vi "FGV_Chrono.vi"(7 "FGV_state":T2, 8 "error in":errorcluster caption="entrée d'erreur", 10 "Taget Time":dbl format="%#_g s") -> (0 "error out":errorcluster caption="sortie d'erreur", 3 "Local":T1 {"Countdown" format="%#_g s"; "Previous Pause TimeTime" format="%#_g s"; "Pause TimeTime" format="%#_g s"; "Time" format="%#_g s"})   [LabVIEW 2020]
doc: "FGV chrono"
uses:
  Controls/Ctrl_states.ctl
  Controls/Ctrl_Local_FGV_Time.ctl
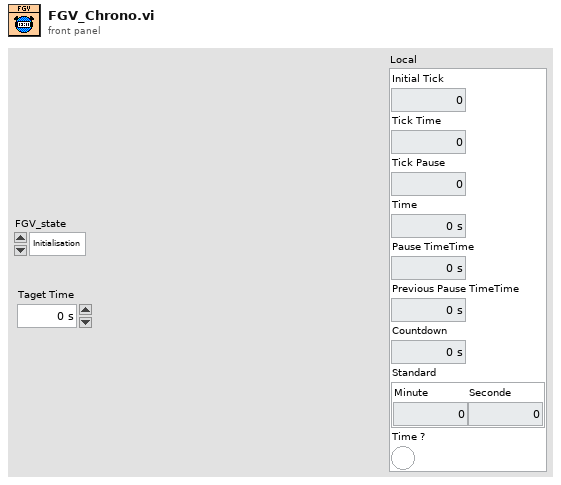
[diagram p1: front panel]
types:
  T1 = typedef "Ctrl_Local_FGV_Time.ctl" = cluster{"Initial Tick":u32, "Tick Time":u32, "Tick Pause":u32, "Time":dbl, "Pause TimeTime":dbl, "Previous Pause TimeTime":dbl, "Countdown":dbl, "Standard":cluster{"Minute":dbl, "Seconde":dbl}, "Time ?":bool}
  T2 = typedef "Ctrl_states.ctl" = enum16{"Initialisation", "Idle", "Stop", "Error", "Display", "Etat 1", "Etat 2", "Etat 3", "Btn_num", "Btn_operator"}
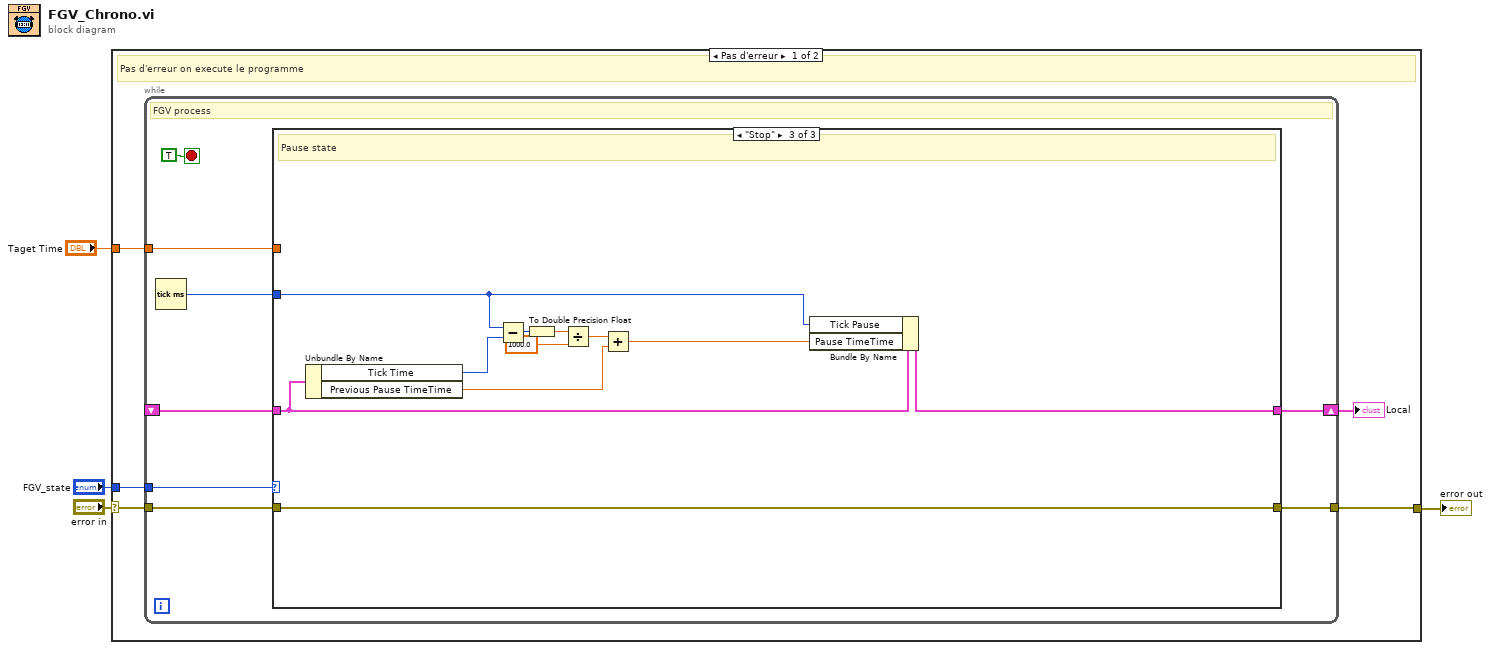
[diagram p0: block diagram]
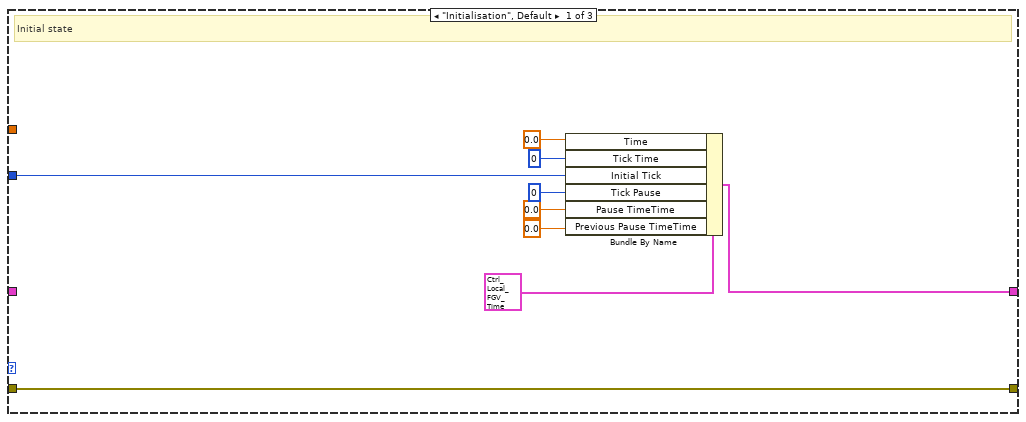
[diagram p2: hidden frame]
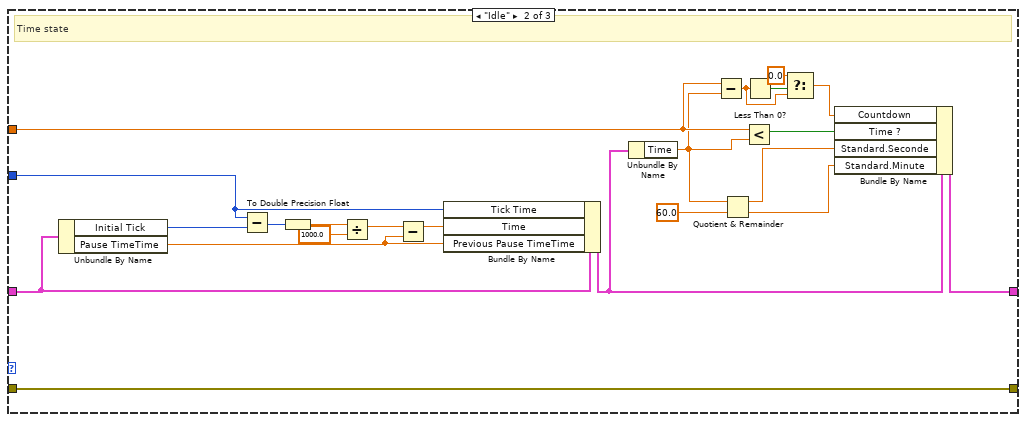
[diagram p3: hidden frame]
diagram:
  n1 = case shown="Pas d'erreur" "error in" {
    selector: "error in" -> [w9 w60]
    tunnel: [w7 w60] -> w3
    tunnel: "FGV_state" -> [w8 _]
    tunnel: "Taget Time" -> [w5 _]
    frame No Error {
      # "Pas d'erreur on execute le programme"
      n2 = while {
        tunnel: w9 -> [w13]
        tunnel: w8 -> [w16]
        shift-right: [w14] -> w6
        shift-left: _ -> [w11]
        tunnel: [w12] -> w7
        tunnel: w5 -> [w10]
        stop <- TRUE stop-if-true
        # "FGV process"
        n3 = Tick Count (ms)() -> (millisecond timer value=w15:u32)
        n4 = case shown="\"Stop\"" w16 {
          tunnel: w15 -> [w24 w41 w49]
          tunnel: [w25 w37 w58] -> w14
          tunnel: w13 -> [w21 w48 w59]
          tunnel: [w21 w48 w59] -> w12
          tunnel: w11 -> [_ w47 w57]
          tunnel: w10 -> [_ w32 _]
          frame "Initialisation", Default {
            # "Initial state"
            n5 = Bundle By Name(cluster=T1 {"Initial Tick"=0, "Tick Time"=0, "Tick Pause"=0, "Time"=0.0, "Pause TimeTime"=0.0, "Previous Pause TimeTime"=0.0, "Countdown"=0.0, "Standard"={"Minute"=0.0, "Seconde"=0.0}, "Time ?"=FALSE} ("Local"), "Time"=0.0, "Tick Time"=u32 0, "Initial Tick"=w24, "Tick Pause"=u32 0, "Pause TimeTime"=0.0, "Previous Pause TimeTime"=0.0) -> (w25:T1)
          }
          frame "Idle" {
            # "Time state"
            n6 = Unbundle By Name(w47) -> ("Initial Tick"=w46:u32, "Pause TimeTime"=w39:dbl)
            n7 = Subtract(x=w41, y=w46) -> (x-y=w45:u32)
            n8 = To Double Precision Float(number=w45) -> (double precision float=w44:dbl)
            n9 = Divide(x=w44, y=1000.0) -> (x/y=w42:dbl)
            n10 = Subtract(x=w42, y=w39) -> (x-y=w40:dbl)
            n11 = Bundle By Name(cluster=w47, "Tick Time"=w41, "Time"=w40, "Previous Pause TimeTime"=w39) -> (w38:T1)
            n12 = Unbundle By Name(w38) -> ("Time"=w31:dbl)
            n13 = Subtract(x=w32, y=w31) -> (x-y=w27:dbl)
            n14 = Quotient & Remainder(x=w31, y=60.0) -> (x-y*floor(x/y)=w34:dbl, floor(x/y)=w33:dbl)
            n15 = Less?(x=w32, y=w31) -> (x < y?=w36:bool)
            n16 = Less Than 0?(x=w27) -> (x < 0?=w30:bool)
            n17 = Select(t=0.0 ("cas vrai"), s=w30, f=w27) -> (s? t:f=w28:dbl)
            n18 = Bundle By Name(cluster=w38, "Countdown"=w28, "Time ?"=w36, "Standard.Seconde"=w34, "Standard.Minute"=w33) -> (w37:T1)
          }
          frame "Stop" {
            # "Pause state"
            n19 = Unbundle By Name(w57) -> ("Tick Time"=w56:u32, "Previous Pause TimeTime"=w51:dbl)
            n20 = Subtract(x=w49, y=w56) -> (x-y=w55:u32)
            n21 = To Double Precision Float(number=w55) -> (double precision float=w54:dbl)
            n22 = Divide(x=w54, y=1000.0) -> (x/y=w52:dbl)
            n23 = Add(x=w52, y=w51) -> (x+y=w50:dbl)
            n24 = Bundle By Name(cluster=w57, "Tick Pause"=w49, "Pause TimeTime"=w50) -> (w58:T1)
          }
        }
      }
      "Local" <- w6
    }
    frame Error {
      # "erreur on laisse passer le flux"
    }
  }
  "error out" <- w3
